vi "Configure Controller.vi"(11 "Config File Path":path=path "TestStand.ini") -> (0 "error IO":errorcluster, 3 "Absolute Path":path)   [LabVIEW 2016, in "TestStand API.lvlib"]
uses:
  TestStand API.lvlib
  MAL-Framework-API/Controller API.lvclass
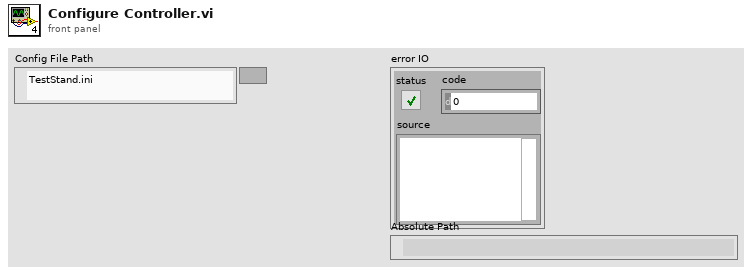
[diagram p1: front panel]
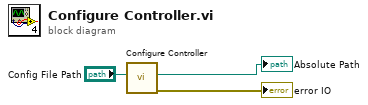
[diagram p0: block diagram]
diagram:
  n1 = call "Configure Controller.vi"("Config File Path"="Config File Path") -> ("error IO"=→"error IO":errorcluster, "Absolute Path"=→"Absolute Path":path)  [unwired: 8 in, 1 out]
